vi "GT Set Laser Crd Map.vi"(8 "error in (no error)":errorcluster caption="错误输入（无错误）", 9 "map":i16, 10 "channel":i16, 11 "cardNum":i16) -> (0 "error out":errorcluster caption="错误输出", 3 "function return":i16)   [LabVIEW 2014, in "gts.lvlib"]
doc: "GT_API GT_SetLaserCrdMap(short cardNum,short channel,short map);"
uses:
  gts.lvlib
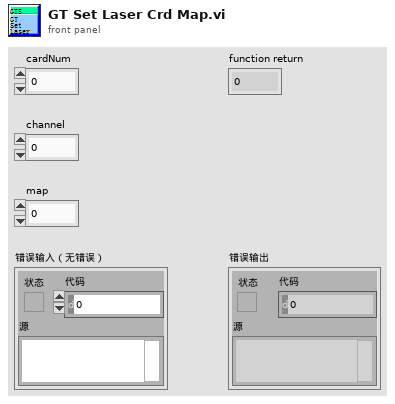
[diagram p1: front panel]
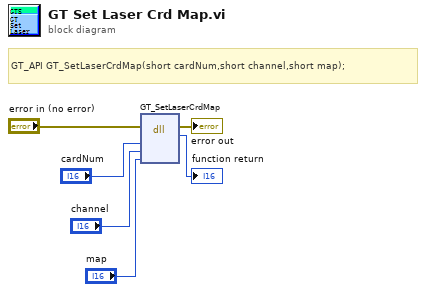
[diagram p0: block diagram]
diagram:
  # "GT_API GT_SetLaserCrdMap(short cardNum,short channel,short map);"
  n1 = dll-call lib="PTH2habs D固高科技资料GTS控制卡GTS卡18年上半年资料dllVC32bit\nmulti_cardgts.*" fn="GT_SetLaserCrdMap"(error in="error in (no error)", "cardNum"="cardNum", "channel"="channel", "map"="map") -> (error out=→"error out":errorcluster, →"function return":i16)  [unwired: 5 in, 1 out]
